vi "RecorderFeed.vi"(4 "Powers Array":i16[](array[numeric])=[0], 5 "Terminate Button":bool, 6 "Enabled?":bool, 7 "NXT":T1={"Hardware"="NXT", "Flattened String"=""}) -> (3 "NXT":T1={"Hardware"="NXT", "Flattened String"=""})   [LabVIEW 2010, in "Recorder.lvlib"]
uses:
  Recorder.lvlib
  <vilib>/NXT/Subs/LVHSConnector.ctl
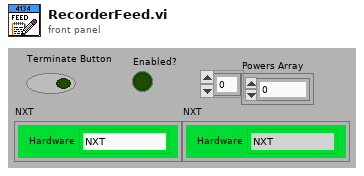
[diagram p1: front panel]
types:
  T1 = typedef "LVHSConnector.ctl" = cluster{"Hardware":string, "Flattened String":string}
  T2 = cluster{"FileName":string, "WriterEnabled?":bool, "TeleopEnabled?":bool, "StopProgram?":bool, "ArraySize":u8}
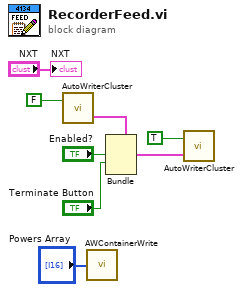
[diagram p0: block diagram]
diagram:
  n1 = call "AutoWriterCluster.vi"("Mode(Write=True)"=FALSE) -> ("Output"=w8:T2)  [unwired: 1 in]
  n2 = call "AWContainerWrite.vi"("Input"="Powers Array") -> ()  [unwired: 1 in]
  n3 = Bundle(cluster=w8, "TeleopEnabled?"="Enabled?", "StopProgram?"="Terminate Button") -> (w7:T2)  [unwired: 3 in]
  n4 = call "AutoWriterCluster.vi"("Mode(Write=True)"=TRUE, "Input"=w7) -> ()  [unwired: 1 out]
  "NXT" <- "NXT"
